vi "main_remote.vi"() -> ()   [LabVIEW 2019]
uses:
  <vilib>/platform/TimedLoop/XDataNode/XDataNode.xnode
  <vilib>/Platform/TimedLoop/XDataNode/nitl_modes.ctl
  <vilib>/Platform/TimedLoop/XDataNode/XDNodeRunTimeDep.lvlib
  <vilib>/Platform/TimedLoop/XDataNode/wakeup.ctl
  <vilib>/Platform/TimedLoop/XDataNode/timing_clust.ctl
  subVI/motor/motor enum.ctl
  sub/servo state.ctl
  <vilib>/myRIO/Express VI/Onboard IO/DO/DO Express VI.xnode
  <vilib>/myRIO/Instrument Drivers/Onboard IO/DIO/vis/Write.vi
  <vilib>/myRIO/Instrument Drivers/Onboard IO/DIO/DIO.lvlib
  <vilib>/myRIO/Common/Instrument Driver Framework/myRIO v1.0/DIO/typedefs/DIO Channels Enum.ctl
  <vilib>/myRIO/Common/Instrument Driver Framework/myRIO v1.0/DIO/typedefs/DIO Channels List.ctl
  <vilib>/myRIO/Common/Instrument Driver Framework/Utilities/typedefs/Generic FPGA Reference.ctl
  <vilib>/myRIO/Common/Instrument Driver Framework/Utilities/typedefs/myRIO v1.0 Reference.ctl
  <vilib>/myRIO/Common/Instrument Driver Framework/Utilities/typedefs/Hardware Version Enum.ctl
  <vilib>/myRIO/Common/Instrument Driver Framework/Utilities/typedefs/myRIO Generic Hardware Reference.ctl
  <vilib>/myRIO/Instrument Drivers/Onboard IO/DIO/typedefs/DIO Reference.ctl
  <vilib>/myRIO/Instrument Drivers/Onboard IO/DIO/vis/myRIO DIO Open.xnode
  <vilib>/myRIO/Common/Instrument Driver Framework/Utilities/vis/Is FPGA Ref Available.vi
  <vilib>/myRIO/Common/Instrument Driver Framework/myRIO v1.0/DIO/vis/myRIO v1.1 Open DIO.vi
  <vilib>/userDefined/High Color/nirio_resource_hc.ctl
  <vilib>/myRIO/Express VI/Onboard Devices/LED/LED Express VI.xnode
  <vilib>/myRIO/Express VI/Onboard Devices/Button/Button Express VI.xnode
  <vilib>/myRIO/Instrument Drivers/Onboard IO/DIO/vis/Read.vi
  <userlib>/KNR OS 4.0 LabVIEW Toolkit/F710/f710.ctl
panel:
  out "F710":T1
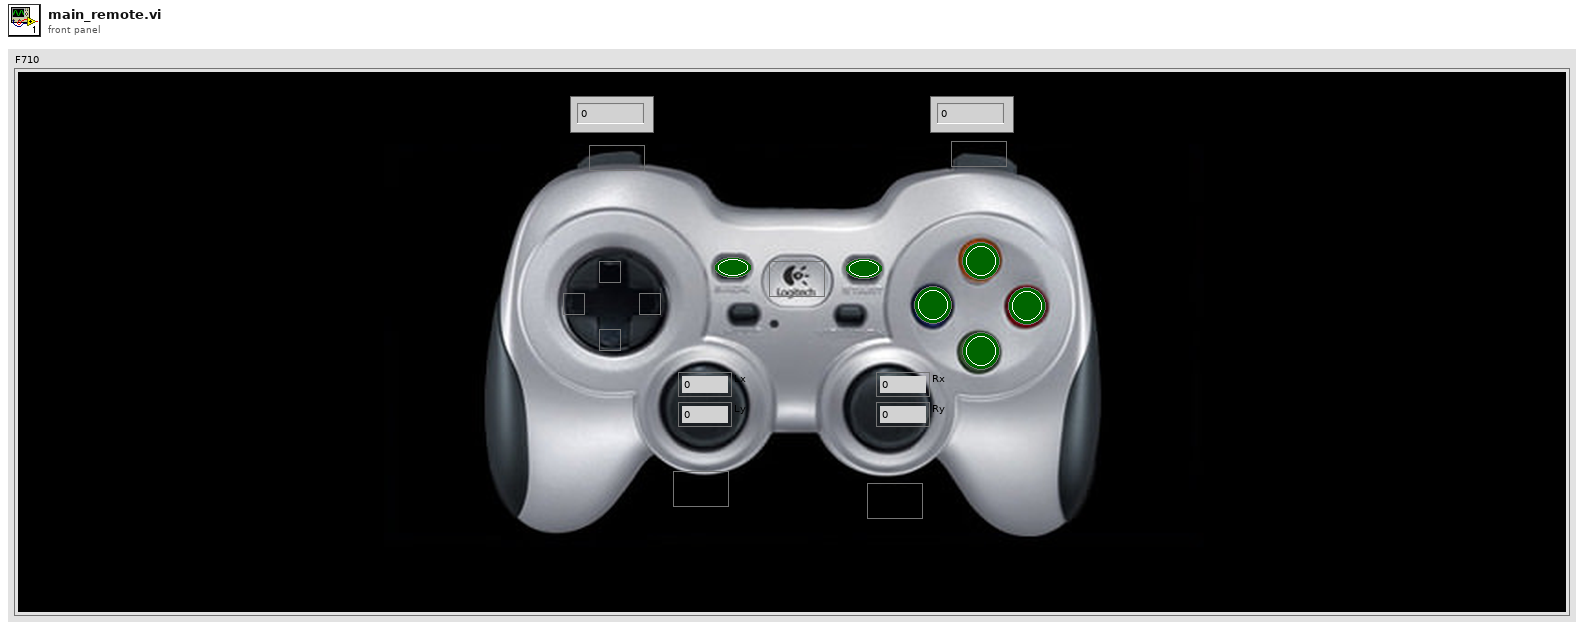
[diagram p1: front panel]
types:
  T1 = typedef "f710.ctl" = cluster{"Down":bool, "Left":bool, "Up":bool, "Right":bool, "A":bool, "X":bool, "Y":bool, "B":bool, "LB":bool, "RB":bool, "LT":i16, "RT":i16, "L3":bool, "R3":bool, "Ly":i16, "Lx":i16, "Ry":i16, "Rx":i16, "Back":bool, "Start":bool, "center":bool}
  T2 = typedef "servo state.ctl" = enum16{"catch", "cam-1", "put", "side", "center", "side-2", "put-2"}
  T3 = typedef "DIO.lvlib/DIO Reference.ctl" = cluster{"myRIO Reference":T4, "DIO Channels List":T8}
  T4 = typedef "myRIO Generic Hardware Reference.ctl" = cluster{"myRIO Model":T5, "myRIO Hardware Reference":T6}
  T5 = typedef "Hardware Version Enum.ctl" = enum16{"Unknown", "myRIO-1900", "myRIO-1950", "roboRIO", "NI ELVIS RIO CM", "ELVIS III"}
  T6 = typedef "myRIO v1.0 Reference.ctl" = cluster{"Generic FPGA Reference":T7, "Allow multiple opens":bool}
  T7 = typedef "Generic FPGA Reference.ctl" = refnum<k20>
  T8 = typedef "DIO Channels List.ctl" = T9[]
  T9 = typedef "DIO Channels Enum.ctl" = enum16{"Not Connected", "C/DIO0", "C/DIO1", "C/DIO2", "C/DIO3", "C/DIO4", "C/DIO5", "C/DIO6", "C/DIO7", "A/DIO0", "A/DIO1", "A/DIO2", "A/DIO3", "A/DIO4", "A/DIO5", "A/DIO6", "A/DIO7", "A/DIO8", "A/DIO9", "A/DIO10", "A/DIO11", "A/DIO12", "A/DIO13", "A/DIO14", "A/DIO15", "A/DIO16", "A/DIO17", "A/DIO18", "A/DIO19", "B/DIO0", "B/DIO1", "B/DIO2", "B/DIO3", "B/DIO4", "B/DIO5", "B/DIO6", "B/DIO7", "B/DIO8", "B/DIO9", "B/DIO10", "B/DIO11", "B/DIO12", "B/DIO13", "B/DIO14", "B/DIO15", "B/DIO16", "B/DIO17", "B/DIO18", "B/DIO19", "LED0", "LED1", "LED2", "LED3", "Button0", "DIO/DIO0", "DIO/DIO1", "DIO/DIO2", "DIO/DIO3", "DIO/DIO4", "DIO/DIO5", "DIO/DIO6", "DIO/DIO7", "DIO/DIO8", "DIO/DIO9", "SPI/CS0", "SPI/CS1", "SPI/CS2", "SPI/CS3", "LED RADIO (Green)", "LED RADIO (Red)", "LED COMM (Green)", "LED COMM (Red)", "LED MODE (Green)", "LED MODE (Red)"}
  T10 = typedef "nirio_resource_hc.ctl" = tag
  T11 = typedef "XDNodeRunTimeDep.lvlib/timing_clust.ctl" = cluster{"Expected End [f-1]":u64, "Actual End [f-1]":u64, "Finished Late? [f-1]":bool, "Expected End [i-1]":u64, "Actual End [i-1]":u64, "Finished Late? [i-1]":bool, "Expected Start [i]":u64, "Actual Start [i]":u64, "Expected Start [f]":u64, "Actual Start [f]":u64, "Source Name":string, "Structure Name":string, "Period":i64, "Deadline":i64, "Offset":i64, "Start":i64, "Priority":i32, "Timeout":i32, "Mode":T12, "Wakeup Reason":T13, "Error":errorcluster, "Source Type":string, "Secondary Source Type":string, "Global End Time":u64, "Global Start Time":u64, "Frame Duration":u64, "Iteration Duration":u64, "Assigned CPU":i32, "I/O Scan Engine Mode":u32}
  T12 = typedef "XDNodeRunTimeDep.lvlib/nitl_modes.ctl" = enum32{"No Change", "Process missed periods, maintain original phase", "Discard missed periods, maintain original phase", "Process missed periods, ignore original phase", "Discard missed periods, ignore original phase"}
  T13 = typedef "XDNodeRunTimeDep.lvlib/wakeup.ctl" = enum32{"Normal", "Aborted", "Asynchronous wakeup", "Timing source error", "Timed loop error", "Timeout"}
  T14 = typedef "motor enum.ctl" = enum16{"M1", "M2", "M3", "M4"}
  T15 = cluster{"proportional gain (Kc)":dbl, "integral time (Ti, min)":dbl, "derivative time (Td, min)":dbl}
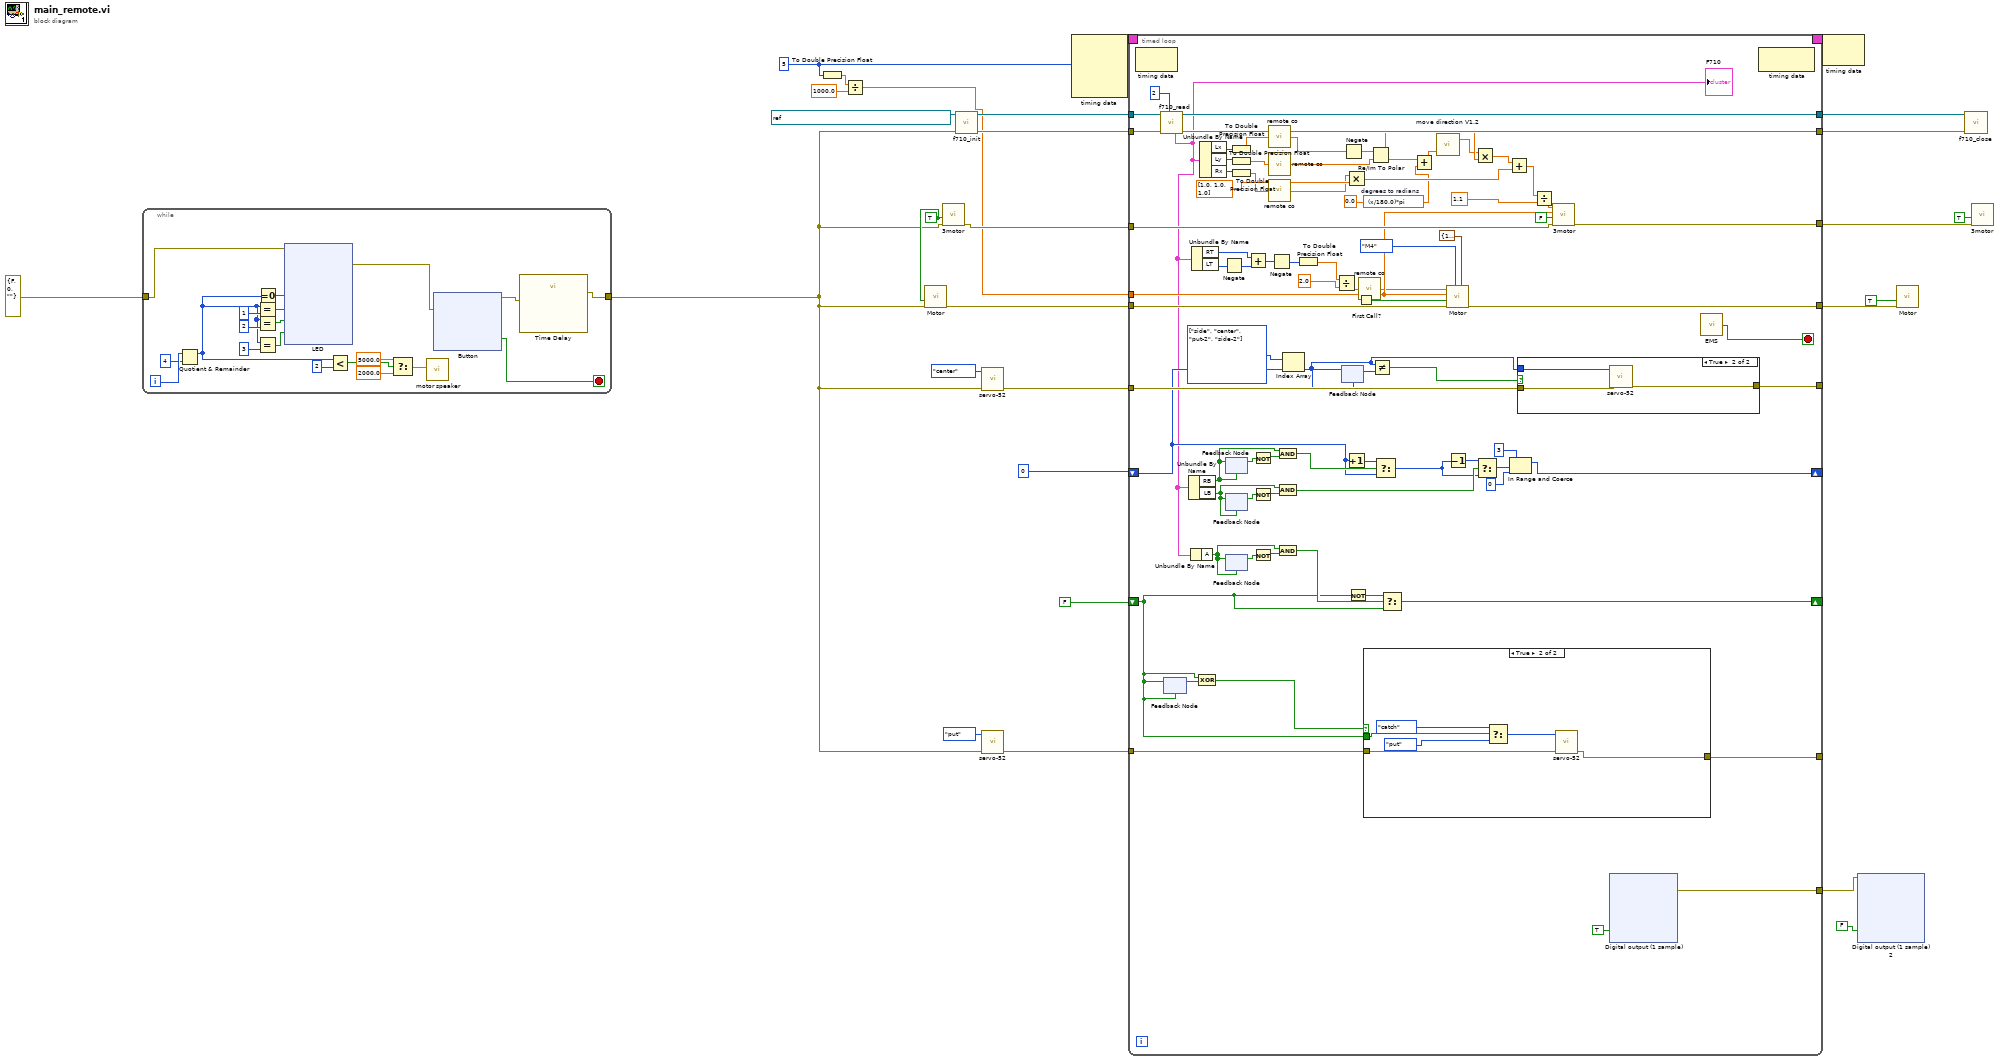
[diagram p0: block diagram]
diagram:
  w18 = i64 5 ("Period")
  w13 = TRUE ("Reset")
  n1 = while {
    tunnel: errorcluster {"status"=FALSE, "code"=0, "source"=""} ("error in (no error)") -> [w39]
    tunnel: [w36] -> w1
    i -> [w48]
    stop <- w37 stop-if-true
    n2 = Quotient & Remainder(x=w48, y=4) -> (x-y*floor(x/y)=w34:i32)  [unwired: 1 out]
    n3 = Equal?(x=w34, y=1) -> (x = y?=w45:bool)
    n4 = Equal?(x=w34, y=2) -> (x = y?=w42:bool)
    n5 = Equal?(x=w34, y=3) -> (x = y?=w41:bool)
    n6 = Equal To 0?(x=w34) -> (x = 0?=w46:bool)
    n7 = xnode "LED"("LED0"=w46, "LED1"=w45, "LED2"=w42, "LED3"=w41, "error in (no error)"=w39) -> ("error out"=w38:errorcluster)
    n8 = Less?(x=w34, y=2) -> (x < y?=w31:bool)
    n9 = Select(t=5000.0, s=w31, f=2000.0) -> (s? t:f=w32:dbl)
    n10 = call "motor speaker.vi"("Vertical Pointer Slide"=w32) -> ()  [unwired: 11 in]
    n11 = xnode "Button"("error in (no error)"=w38) -> ("Value"=w37:bool, "error out"=w35:errorcluster)
    n12 = call "Time Delay"("error in (no error)"=w35) -> ("error out"=w36:errorcluster)  [unwired: 10 in]
  }
  n13 = To Double Precision Float(number=w18) -> (double precision float=w17:dbl)
  n14 = Divide(x=w17, y=1000.0) -> (x/y=w15:dbl)
  n15 = call "Motor.vi"("error in (no error)"=w1, "Reset"=w13) -> ("error out"=w14:errorcluster)  [unwired: 6 in, 3 out]
  n16 = call "3motor.vi"("error in (no error)"=w1, "Reset"=w13) -> ("error out"=w19:errorcluster)  [unwired: 8 in, 1 out]
  n17 = call <userlib>:"f710_init.vi"("error in (no error)"=w1, "USB RAW VISA resource name"=refnum<visa-resource-name> "USB0::0x046D::0xC21F::EEAB948F::RAW") -> ("error out"=w25:errorcluster, "VISA Refnum out"=w24:refnum<visa-resource-name>)  [unwired: 8 in]
  n18 = call "servo-52.vi"("error in (no error)"=w1, "Enum"=servo_state."center") -> ("error out"=w9:errorcluster)  [unwired: 9 in]
  n19 = call "servo-52.vi"("error in (no error)"=w1, "Enum"=servo_state."put") -> ("error out"=w6:errorcluster)  [unwired: 9 in]
  n20 = node-c288(w18) -> (w28:T11)  [unwired: 3 in]
  n21 = timed-loop {
    timing: w28 -> [_]
    timing-out: [_] -> w27
    tunnel: [w203] -> w26
    tunnel: w25 -> [w202]
    tunnel: w24 -> [w201]
    tunnel: [w200] -> w23
    tunnel: [w193] -> w21
    tunnel: w19 -> [w191]
    tunnel: w15 -> [w176]
    tunnel: w14 -> [w175]
    tunnel: [w174] -> w12
    shift-right: [w154] -> _
    shift-left: 0 -> [w159]
    tunnel: w9 -> [w170]
    tunnel: [w150] -> _
    shift-right: [w143] -> _
    shift-left: FALSE -> [w139]
    tunnel: w6 -> [w140]
    tunnel: [w138] -> _
    tunnel: [w135] -> w4
    stop <- w185 stop-if-true
    w171 = T2[] [enum."side", enum."center", enum."put-2", enum."side-2"] items=["catch", "cam-1", "put", "side", "center", "side-2", "put-2"] ("Array")
    n22 = node-c288() -> ()  [unwired: 1 in, 1 out]
    n23 = call <userlib>:"f710_read.vi"("Timeout to wait for Interrupt (ms)"=u32 2, "error in (no error)"=w202, "VISA Refnum in"=w201) -> ("error out"=w203:errorcluster, "VISA Refnum out"=w200:refnum<visa-resource-name>, "F710"=w149:T1)  [unwired: 6 in]
    "F710" <- w149
    n24 = feedback-in #1(w139) -> ()
    n25 = feedback #1(w139) -> (w142:bool)
    n26 = Unbundle By Name(w149) -> ("RB"=w167:bool, "LB"=w164:bool)
    n27 = Unbundle By Name(w149) -> ("A"=w146:bool)
    n28 = Unbundle By Name(w149) -> ("RT"=w181:i16, "LT"=w183:i16)
    n29 = Exclusive Or(1:w142, 2:w139) -> (0:w141:bool)
    n30 = Unbundle By Name(w149) -> ("Lx"=w199:i16, "Ly"=w198:i16, "Rx"=w197:i16)
    n31 = Negate(x=w183) -> (-x=w182:i16)
    n32 = feedback-in #2(w167) -> ()
    n33 = feedback #2(w167) -> (w168:bool)
    n34 = feedback #3(w164) -> (w166:bool)
    n35 = feedback-in #3(w164) -> ()
    n36 = feedback #4(w146) -> (w147:bool)
    n37 = feedback-in #4(w146) -> ()
    n38 = To Double Precision Float(number=w199) -> (double precision float=w133:dbl)
    n39 = To Double Precision Float(number=w198) -> (double precision float=w131:dbl)
    n40 = To Double Precision Float(number=w197) -> (double precision float=w128:dbl)
    n41 = Add(x=w181, y=w182) -> (x+y=w180:i16)
    n42 = Not(x=w168) -> (.not. x?=w169:bool)
    n43 = Not(x=w166) -> (.not. x?=w165:bool)
    n44 = Not(x=w147) -> (.not. x?=w148:bool)
    n45 = call "remote co.vi"("input"=w133) -> ("x*y"=w132:dbl)
    n46 = call "remote co.vi"("input"=w131) -> ("x*y"=w130:dbl)
    n47 = call "remote co.vi"("input"=w128) -> ("x*y"=w129:dbl)
    n48 = Negate(x=w180) -> (-x=w177:i16)
    n49 = And(x=w167, y=w169) -> (x .and. y?=w163:bool)
    n50 = And(x=w164, y=w165) -> (x .and. y?=w161:bool)
    n51 = And(x=w146, y=w148) -> (x .and. y?=w145:bool)
    n52 = Index Array(array=w171, index=w159) -> (element=w151:T2)
    n53 = To Double Precision Float(number=w177) -> (double precision float=w127:dbl)
    n54 = Divide(x=w127, y=2.0) -> (x/y=w173:dbl)
    n55 = feedback #5(w151) -> (w153:T2)
    n56 = feedback-in #5(w151) -> ()
    n57 = Negate(x=w132) -> (-x=w184:dbl)
    n58 = Multiply(x=w129, y=dbl[] [1.0, 1.0, 1.0]) -> (x*y=w194:dbl[])
    n59 = Increment(x=w159) -> (x+1=w160:i32)
    n60 = Not(x=w139) -> (.not. x?=w144:bool)
    n61 = First Call?() -> (First Call?: T/F=w137:bool)
    n62 = call "remote co.vi"("input"=w173) -> ("x*y"=w126:dbl)
    n63 = expression code="(x/180.0)*pi" "degrees to radians"(0.0) -> (w124:dbl)
    n64 = case shown="True" w141 {
      tunnel: w140 -> [w239 w245]
      tunnel: w139 -> [_ w244]
      tunnel: [w239 w240] -> w138
      frame False {
      }
      frame True {
        n65 = Select(t=servo_state."catch" ("Enum"), s=w244, f=servo_state."put" ("Enum")) -> (s? t:f=w241:T2)
        n66 = call "servo-52.vi"("error in (no error)"=w245, "Enum"=w241) -> ("error out"=w240:errorcluster)  [unwired: 9 in]
      }
    }
    n67 = Re/Im To Polar(2:w130, 3:w184) -> (0:w125:dbl, 1:w188:dbl)
    n68 = Not Equal?(x=w151, y=w153) -> (x != y?=w152:bool)
    n69 = Select(t=w160, s=w163, f=w159) -> (s? t:f=w158:i32)
    n70 = Select(t=w144, s=w145, f=w139) -> (s? t:f=w143:bool)
    n71 = Add(x=w125, y=w124) -> (x+y=w123:dbl)
    n72 = call "move direction V1.2.vi"("theta"=w123) -> ("out array"=w187:dbl[])  [unwired: 1 in, 1 out]
    n73 = call "Motor.vi"("PID gains"=T15 {"proportional gain (Kc)"=10.0, "integral time (Ti, min)"=0.0, "derivative time (Td, min)"=0.0002}, "Enum"=motor_enum."M4", "error in (no error)"=w175, "Reset"=w137, "dt(s)"=w176, "RPM"=w126) -> ("error out"=w174:errorcluster)  [unwired: 2 in, 3 out]
    n74 = Decrement(x=w158) -> (x-1=w162:i32)
    n75 = Multiply(x=w187, y=w188) -> (x*y=w195:dbl[])
    n76 = Select(t=w162, s=w161, f=w158) -> (s? t:f=w157:i32)
    n77 = Add(x=w195, y=w194) -> (x+y=w136:dbl[])
    n78 = In Range and Coerce(upper limit=3, x=w157, lower limit=0) -> (coerced(x)=w154:i32)  [unwired: 1 out]
    n79 = case shown="True" w152 {
      tunnel: w151 -> [_ w249]
      tunnel: w170 -> [w246 w248]
      tunnel: [w246 w247] -> w150
      frame False {
      }
      frame True {
        n80 = call "servo-52.vi"("error in (no error)"=w248, "Enum"=w249) -> ("error out"=w247:errorcluster)  [unwired: 9 in]
      }
    }
    n81 = Divide(x=w136, y=1.1) -> (x/y=w190:dbl[])
    n82 = call "3motor.vi"("error in (no error)"=w191, "Reset"=FALSE, "dt(s)"=w176, "Motor speed"=w190) -> ("error out"=w193:errorcluster)  [unwired: 6 in, 1 out]
    n83 = xnode "Digital output (1 sample)"("C/DIO1 (DIO1)"=TRUE ("C/DIO5 (DIO5)")) -> ("error out"=w135:errorcluster)  [unwired: 1 in]
    n84 = call "EMS.vi"() -> ("A/DIO4 (Pin 19)"=w185:bool)
    n85 = node-c288() -> ()  [unwired: 1 in, 1 out]
  }
  n86 = node-c288(w27) -> ()  [unwired: 1 out]
  n87 = xnode "Digital output (1 sample) 2"("C/DIO1 (DIO1)"=FALSE ("C/DIO5 (DIO5)"), "error in (no error)"=w4) -> ()  [unwired: 1 out]
  n88 = call "Motor.vi"("error in (no error)"=w12, "Reset"=TRUE) -> ()  [unwired: 6 in, 4 out]
  n89 = call <userlib>:"f710_close.vi"("error in (no error)"=w26, "VISA Refnum in"=w23) -> ()  [unwired: 9 in, 1 out]
  n90 = call "3motor.vi"("error in (no error)"=w21, "Reset"=TRUE) -> ()  [unwired: 8 in, 2 out]
